vi "Read Scaling coefficients.vi"(8 "error in (no error)":errorcluster, 11 "NI-Scope Lock-in Driver in":refnum<class "NI-Scope Lock-in Driver.lvclass">) -> (0 "error out":errorcluster, 2 "Scaling coefficients":dbl[][](array[numeric]), 3 "NI-Scope Lock-in Driver out":refnum<class "NI-Scope Lock-in Driver.lvclass">)   [LabVIEW 2016, in "NI-Scope Lock-in Driver.lvclass"]
uses:
  NI-Scope Lock-in Driver.lvclass
  NI-Scope Digitizer/Ni-Scope Digitizer.lvclass
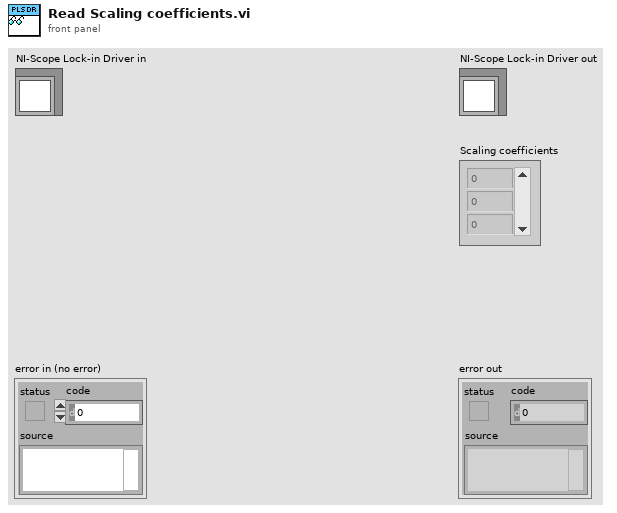
[diagram p1: front panel]
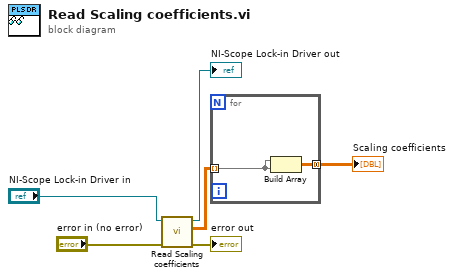
[diagram p0: block diagram]
diagram:
  n1 = call-parent "Read Scaling coefficients.vi"("error in (no error)"="error in (no error)", "Pulse Driver in"="NI-Scope Lock-in Driver in") -> ("error out"=→"error out":errorcluster, "Scaling coefficients"=w2:dbl[][], "Pulse Driver out"=→"NI-Scope Lock-in Driver out":refnum<class "NI-Scope Lock-in Driver.lvclass">)  [unwired: 7 in]
  n2 = for {
    tunnel: w2 -> [w8] mode=indexing
    tunnel: [w7] -> w1 mode=concatenating
    n3 = Build Array(w8, w8) -> (w7:dbl[][])
  }
  "Scaling coefficients" <- w1
